vi "Load from INI.vi"(8 "error in (no error)":errorcluster, 10 "INI Path":path, 11 "HAL Manager in":refnum<class "HAL Manager.lvclass">) -> (0 "error out":errorcluster, 3 "HAL Manager out":refnum<class "HAL Manager.lvclass">)   [LabVIEW 2012, in "HAL.lvlib" / "HAL Manager.lvclass"]
doc: "Use this VI to load devices and configuration saved in the specified INI file. INI files should be generated using the Save to INI VI on this class which is the same method used by the configuration editor.\n\nIf an existing Manager instance is not wired into the VI, a new instance will be created for the devices to be added to and then that instance will be returned. Wiring in an existing Manager instance will have the loaded devices added to existing devices managed by that instance."
uses:
  HAL Manager.lvclass
  <vilib>/Utility/config.llb/NI_LVConfig.lvlib
  Device Config.ctl
  <vilib>/Utility/config.llb/Read Key (Path).vi
  <vilib>/Utility/config.llb/Read Key (String).vi
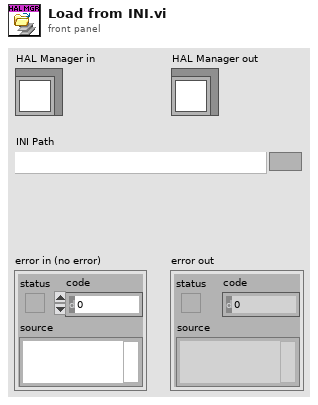
[diagram p1: front panel]
types:
  T1 = typedef "NI_LVConfig.lvlib/Config Data RefNum.ctl" = refnum<k1>
  T2 = typedef "HAL.lvlib/HAL Manager.lvclass/Device Config.ctl" = cluster{"Name":string, "Keys":string[], "Values":string[], "Path":path}
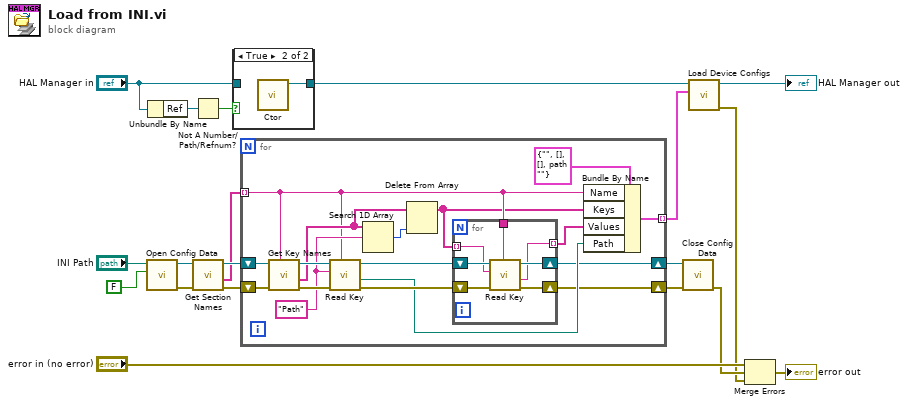
[diagram p0: block diagram]
diagram:
  n1 = call <vilib>:"Open Config Data.vi"("create file if necessary (T)"=FALSE, "configuration file path"="INI Path") -> ("error out"=w15:errorcluster, "refnum"=w16:T1)  [unwired: 7 in, 1 out]
  n2 = Unbundle By Name("HAL Manager in") -> ("Ref"=w4:refnum<data-value>)
  n3 = Not A Number/Path/Refnum?(number/path/refnum=w4) -> (NaN/Path/Refnum?=w3:bool)
  n4 = call <vilib>:"Get Section Names.vi"("error in (no error)"=w15, "refnum"=w16) -> ("error out"=w14:errorcluster, "section names"=w12:string[], "refnum out"=w13:T1)  [unwired: 7 in]
  n5 = case shown="True" w3 {
    tunnel: "HAL Manager in" -> [w20 _]
    tunnel: [w20 w21] -> w1
    frame False {
    }
    frame True {
      n6 = call "Ctor.vi"() -> ("HAL Manager out"=w21:refnum<class "HAL Manager.lvclass">)  [unwired: 10 in, 1 out]
    }
  }
  n7 = for {
    shift-right: [w23] -> w10
    shift-left: w14 -> [w37]
    shift-right: [w24] -> w11
    shift-left: w13 -> [w38]
    tunnel: w12 -> [w28] mode=indexing
    tunnel: [w22] -> w9 mode=indexing
    w34 = "Path"
    n8 = call <vilib>:"Get Key Names.vi"("section"=w28, "error in (no error)"=w37, "refnum"=w38) -> ("error out"=w35:errorcluster, "key names"=w32:string[], "refnum out"=w36:T1)  [unwired: 5 in, 1 out]
    n9 = call-poly <vilib>:"Read Key.vi"("section"=w28, "error in (no error)"=w35, "key"=w34, "refnum"=w36) -> ("error out"=w30:errorcluster, "value"=w25:path, "refnum out"=w31:T1)  [unwired: 4 in, 1 out]
    n10 = Search 1D Array(1D array=w32, element=w34) -> (index of element=w33:i32)  [unwired: 1 in]
    n11 = Delete From Array(array=w32, index=w33) -> (array with subset deleted=w27:string[])  [unwired: 1 in, 1 out]
    n12 = for {
      shift-right: [w41] -> w24
      shift-left: w31 -> [w44]
      shift-right: [w40] -> w23
      shift-left: w30 -> [w45]
      tunnel: w27 -> [w43] mode=indexing
      tunnel: w28 -> [w42]
      tunnel: [w39] -> w26 mode=indexing
      n13 = call-poly <vilib>:"Read Key.vi"("section"=w42, "error in (no error)"=w45, "key"=w43, "refnum"=w44) -> ("error out"=w40:errorcluster, "value"=w39:string, "refnum out"=w41:T1)  [unwired: 4 in, 1 out]
    }
    n14 = Bundle By Name(cluster=T2 {"Name"="", "Keys"=[], "Values"=[], "Path"=path ""} ("Device Config"), "Name"=w28, "Keys"=w27, "Values"=w26, "Path"=w25) -> (w22:T2)
  }
  n15 = call <vilib>:"Close Config Data.vi"("error in (no error)"=w10, "refnum"=w11) -> ("error out"=w6:errorcluster)  [unwired: 8 in, 1 out]
  n16 = call "Load Device Configs.vi"("Device Configs"=w9, "HAL Manager in"=w1) -> ("error out"=w5:errorcluster, "HAL Manager out"=→"HAL Manager out":refnum<class "HAL Manager.lvclass">)  [unwired: 8 in]
  n17 = Merge Errors("error in (no error)", w6, w5) -> (→"error out":errorcluster)
